vi "SignalGenerator.vi"(9 "Stop":bool, 10 "Amplitude (V)":dbl, 11 "Frequency (Hz)":dbl) -> ()   [LabVIEW 2014]
panel:
  out "error out":errorcluster
  out "Sine error out":errorcluster caption="error out"
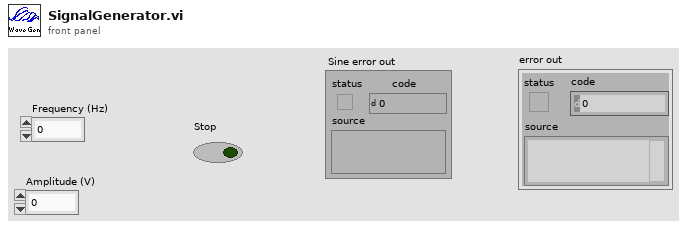
[diagram p1: front panel]
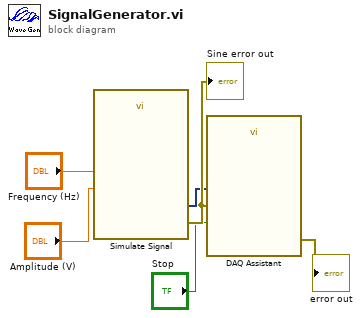
[diagram p0: block diagram]
diagram:
  n1 = call "Simulate Signal"("Frequency"="Frequency (Hz)", "Amplitude"="Amplitude (V)") -> ("Sine"=w2:dynamicdata, "error out"=w4:errorcluster)  [unwired: 12 in]
  "Sine error out" <- w4
  n2 = call "DAQ Assistant"("data"=w2, "error in"=w4, "stop (T)"="Stop") -> ("error out"=→"error out":errorcluster)  [unwired: 15 in, 1 out]
